vi "Read U32.vi"(8 "error in (no error)":errorcluster, 11 "Section 2a in":refnum<class "Section 2a.lvclass">) -> (0 "error out":errorcluster, 2 "U32":u32, 3 "Section 2a out":refnum<class "Section 2a.lvclass">)   [LabVIEW 2012, in "LVOOP Introduction.lvlib" / "Section 2a.lvclass"]
uses:
  Section 2a.lvclass
  Section 2a.lvclass/Section 2a.ctl
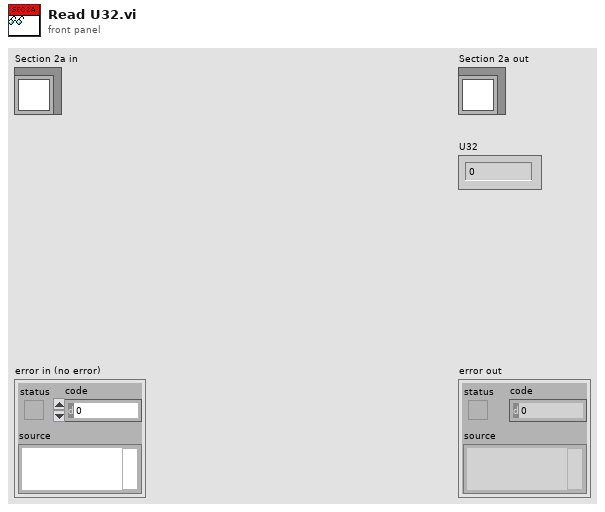
[diagram p1: front panel]
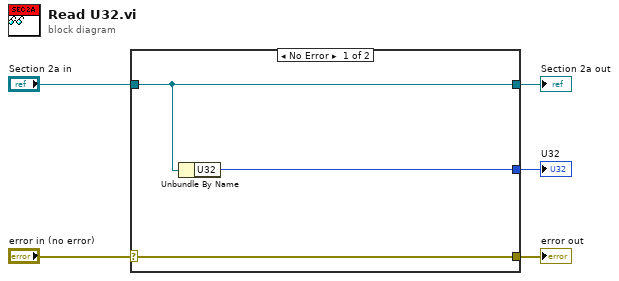
[diagram p0: block diagram]
diagram:
  n1 = case shown="No Error" "error in (no error)" {
    selector: "error in (no error)" -> [w8 w9]
    tunnel: [w8 w9] -> w4
    tunnel: [w7 w10] -> w2
    tunnel: "Section 2a in" -> [w7 w10]
    tunnel: [w6 _] -> w1
    frame No Error {
      n2 = Unbundle By Name(w7) -> ("U32"=w6:u32)
    }
    frame Error {
    }
  }
  "error out" <- w4
  "Section 2a out" <- w2
  "U32" <- w1
